vi "Get Project Path from App Ref.vi"(8 "error in (no error)":errorcluster, 11 "App Ref":refnum<vi>) -> (0 "error out":errorcluster, 2 "Project Path":path, 3 "App Ref out":refnum<vi>)   [LabVIEW 2020, in "MacroAssert.lvlib"]
doc: "Gets the project path for <B>App Ref</B> if it is an application reference whose context is a project in the development system. Outputs an empty path in every other type of context."
uses:
  MacroAssert.lvlib
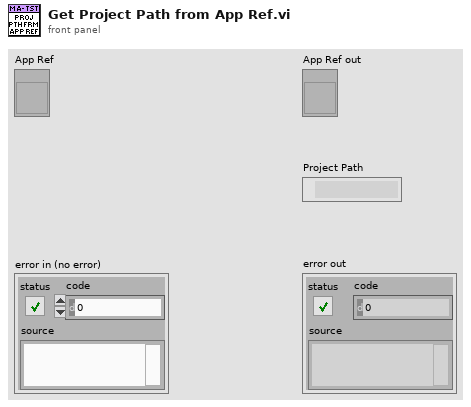
[diagram p1: front panel]
types:
  T1 = enum32{"invalid app kind", "Development System", "Run Time System", "Student Edition", "Embedded LabVIEW", "Evaluation", "Custom"}
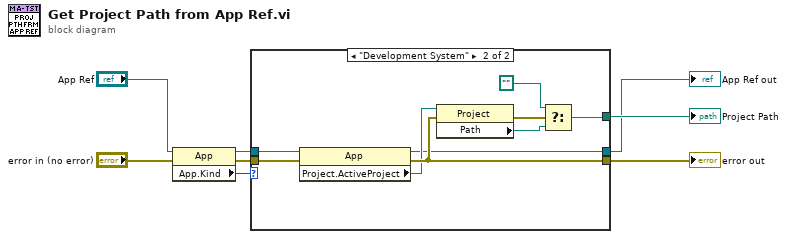
[diagram p0: block diagram]
diagram:
  n1 = property class="App"(reference="App Ref", error in="error in (no error)") -> (reference out=w5:refnum<vi>, error out=w8:errorcluster, "App.Kind"=w3:T1)
  n2 = case shown="\"Development System\"" w3 {
    tunnel: w5 -> [w9 w16]
    tunnel: [_ w11] -> w2
    tunnel: [w9 w14] -> w1
    tunnel: w8 -> [w10 w18]
    tunnel: [w10 w17] -> w6
    frame "invalid app kind", Default {
    }
    frame "Development System" {
      n3 = property class="App"(reference=w16, error in=w18) -> (reference out=w14:refnum<vi>, error out=w17:errorcluster, "Project.ActiveProject"=w15:refnum<vi>)
      n4 = property class="Project"(reference=w15, error in=w17) -> (error out=w19:errorcluster, "Path"=w13:path)  [unwired: 1 out]
      n5 = Select(t=path "", s=w19, f=w13) -> (s? t:f=w11:path)
    }
  }
  "App Ref out" <- w1
  "error out" <- w6
  "Project Path" <- w2
